vi "Unregister For Event.vi"(8 "Error In":errorcluster, 9 "Event Name":string, 10 "Registrant Address":refnum<class "Message Enqueuer.lvclass">, 11 "Event Source Actor In":refnum<class "Event Source Actor.lvclass">) -> (0 "Error Out":errorcluster, 3 "Event Source Actor Out":refnum<class "Event Source Actor.lvclass">)   [LabVIEW 2021, in "EventSourceActor.lvlib" / "Event Source.lvlib" / "Event Source Actor.lvclass"]
doc: "This method unregisters a specific Actors Enqueuer from specific Event he is listening to, in this Event Source Actor."
uses:
  Event Source Actor.lvclass
  <vilib>/ActorFramework/Message Enqueuer/Message Enqueuer.lvclass
  Event Source Actor.lvclass/Event Source Actor.ctl
  c8cb1f89-adbf-4be7-8ea2-29bcf479b04f.vi
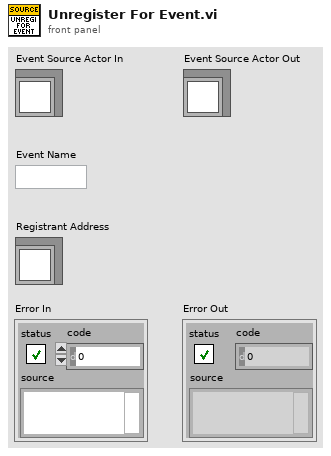
[diagram p1: front panel]
types:
  T1 = map{string, set{refnum<class "Message Enqueuer.lvclass">}}
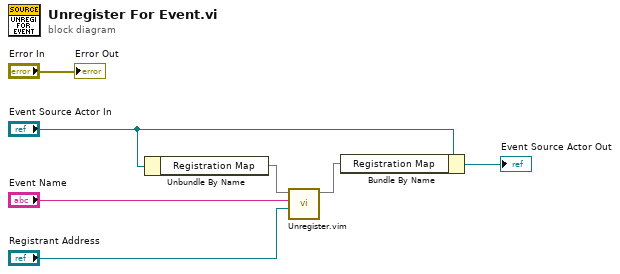
[diagram p0: block diagram]
diagram:
  n1 = Unbundle By Name("Event Source Actor In") -> ("Registration Map"=w7:T1)
  n2 = call "Unregister.vim"("set element"="Registrant Address", "key"="Event Name", "map in"=w7) -> ("map out"=w3:T1)  [unwired: 6 in, 2 out]
  n3 = Bundle By Name(cluster="Event Source Actor In", "Registration Map"=w3) -> (→"Event Source Actor Out":refnum<class "Event Source Actor.lvclass">)
  "Error Out" <- "Error In"
